vi "Drive Globals.vi"() -> ()   [LabVIEW 2017]
uses:
  Drive Notifier.ctl
  Drive Control Type.ctl
panel:
  in  "Robot Distance":dbl
  out "Zero XY?":bool
  out "X position":dbl
  out "Y position":dbl
  in  "Drive Cals":dbl[](array[numeric])
  in  "Robot Heading":dbl
  in  "Drive Execute Notifier":refnum<notifier>
  in  "Drive Set Notifier":refnum<notifier>
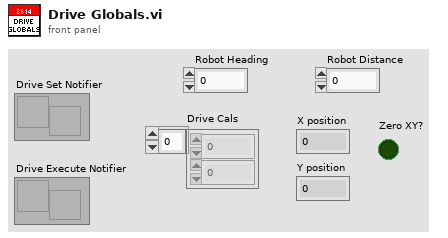
[diagram p1: front panel]
diagram:
